vi "Forward Pass (RNN).vi"(2 "params":T2={"Wxh"=[[0.57813, 2.5697, -0.0219857], [-2.4696, -0.172737, 2.44961362]], "Whh"=[[-1.39960002, 0.96174453], [0.36456552, -0.47706397]], "bh"=[[0.5353143], [-1.98598657]], "Why"=[[-0.6486, 0.76469], [-1.77899, 0.38803572], [-0.1309121, -0.333988]], "by"=[[-0.52841737], [-0.44032028], [-0.8844819]]}, 3 "h[t-1]":T1=[[0.0], [0.0]], 4 "x[t]":T1=[[0.0], [1.0], [0.0]]) -> (0 "p[t]":T1=[[0.20283716485987413], [0.10368793196933078], [0.6934749031707951]], 1 "h[t]":T1=[[0.9959896974183432], [-0.973683146441647]])   [LabVIEW 2014]
uses:
  <vilib>/Analysis/Matrix/Datatypes/RealMatrix.ctl
  <vilib>/Analysis/baseanly.llb/Real A x B.vi
  <vilib>/Analysis/Matrix/Numeric/Add/Add - RM,RM.vi
  <vilib>/Analysis/NI_AALBase.lvlib
  <vilib>/Analysis/Matrix/NI_Matrix.lvlib
panel:
  out "Whx * x[t] + Whh * h[t-1] + bh":T1=[[0.5353143], [-1.98598657]]
  out "Why * h[t]":T1=[[-1.3905646829980003], [-2.1496795525916084], [0.1948113838463529]]
  out "Wxh * x[t]":T1=[[2.5697], [-0.172737]]
  out "y[t] = Why * h[t] + by":T1=[[-1.9189820529980004], [-2.5899998325916083], [-0.6896705161536472]]
  out "sum":dbl=0.7235176863832331
  out "e^y[t]":T1=[[0.14675627623195056], [0.07502005264431227], [0.5017413575069702]]
  out "Whh * h[t-1]":T1
  # "IN"
  # "tanh"
  # "--------->"
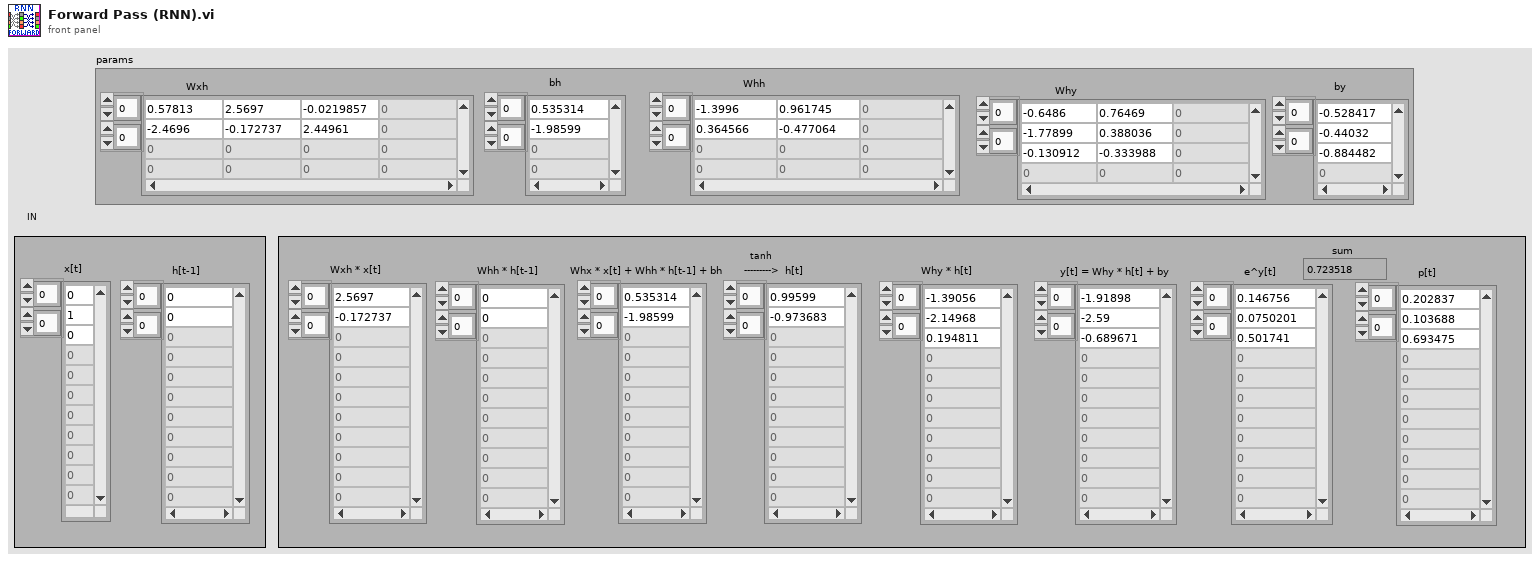
[diagram p1: front panel]
types:
  T1 = typedef "NI_Matrix.lvlib/RealMatrix.ctl" = dbl[][]
  T2 = cluster{"Wxh":T1, "Whh":T1, "bh":T1, "Why":T1, "by":T1}
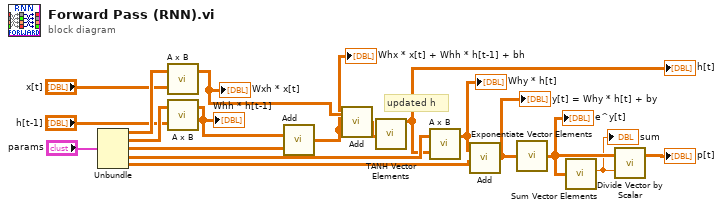
[diagram p0: block diagram]
diagram:
  # "updated h"
  n1 = Unbundle("params") -> ("Wxh"=w14:T1, "Whh"=w15:T1, "bh"=w18:T1, "Why"=w17:T1, "by"=w16:T1)
  n2 = call-poly <vilib>:"A x B.vi"("B"="x[t]", "A"=w14) -> ("A x B"=w6:T1)  [unwired: 1 out]
  "Wxh * x[t]" <- w6
  n3 = call-poly <vilib>:"A x B.vi"("B"="h[t-1]", "A"=w15) -> ("A x B"=w2:T1)  [unwired: 1 out]
  "Whh * h[t-1]" <- w2
  n4 = call-poly <vilib>:"Add.vi"("Real Matrix B"=w18, "Real Matrix A"=w2) -> ("A + B"=w1:T1)
  "Whx * x[t] + Whh * h[t-1] + bh" <- w1
  n5 = call-poly <vilib>:"Add.vi"("Real Matrix B"=w1, "Real Matrix A"=w6) -> ("A + B"=w8:T1)
  n6 = call "TANH Vector Elements.vi"("X"=w8) -> ("tanh(X)"=w9:T1)  [unwired: 18 in]
  "h[t]" <- w9
  n7 = call-poly <vilib>:"A x B.vi"("B"=w9, "A"=w17) -> ("A x B"=w7:T1)  [unwired: 1 out]
  "Why * h[t]" <- w7
  n8 = call-poly <vilib>:"Add.vi"("Real Matrix B"=w16, "Real Matrix A"=w7) -> ("A + B"=w10:T1)
  "y[t] = Why * h[t] + by" <- w10
  n9 = call "Exponentiate Vector Elements.vi"("X"=w10) -> ("exp(X)"=w5:T1)
  "e^y[t]" <- w5
  n10 = call "Sum Vector Elements.vi"("A x B"=w5) -> ("Numeric"=w4:dbl)
  "sum" <- w4
  n11 = call "Divide Vector by Scalar.vi"("Vector"=w5, "x"=w4) -> ("Scaled Vector"=→"p[t]":T1)  [unwired: 17 in]
